vi "Send Inline Buffer.vi"(8 "error in (no error)":errorcluster, 10 "Inline Buffer Parameters":T1, 11 "Dispatcher Interface in":refnum<class "Dispatcher Interface.lvclass">) -> (0 "error out":errorcluster, 3 "Dispatcher Interface out":refnum<class "Dispatcher Interface.lvclass">)   [LabVIEW 2017, in "DSF Core.lvlib" / "Dispatcher Interface.lvclass"]
uses:
  Dispatcher Interface.lvclass
  Inline Buffer Parameters.ctl
  Command Data.ctl
  Command.ctl
  Parameters.ctl
  Write Dispatcher Command.vi
  Interface.lvclass
  Response.ctl
  C:/Git/DSF/Core/Classes/Interface/Interface.lvclass
  Invalid Response.vi
  Invalid Response Parameters.vi
  Read Dispatcher Response.vi
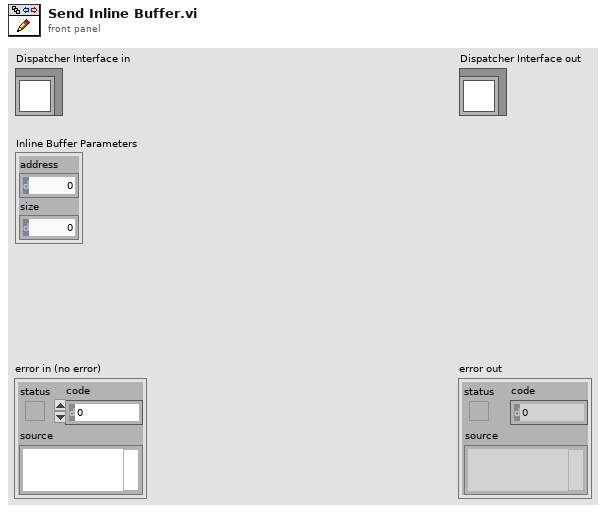
[diagram p1: front panel]
types:
  T1 = typedef "DSF Core.lvlib/Dispatcher Interface.lvclass/Inline Buffer Parameters.ctl" = cluster{"address":u64, "size":u64}
  T2 = typedef "DSF Core.lvlib/Dispatcher Interface.lvclass/Command.ctl" = enum8{"Idle", "Start", "Rx", "Tx", "Set Inline Buffer", "Shutdown", "Error"}
  T3 = typedef "DSF Core.lvlib/Dispatcher Interface.lvclass/Parameters.ctl" = cluster{"arg1":u64, "arg2":u64}
  T4 = typedef "DSF Core.lvlib/Dispatcher Interface.lvclass/Command Data.ctl" = cluster{"Command":T2, "Parameters":T3}
  T5 = typedef "DSF Core.lvlib/Dispatcher Interface.lvclass/Response.ctl" = enum8{"General Ack", "Error", "Shutting Down"}
  T6 = typedef "DSF Core.lvlib/Dispatcher Interface.lvclass/Response Data.ctl" = cluster{"Response":T5, "Parameters":T3}
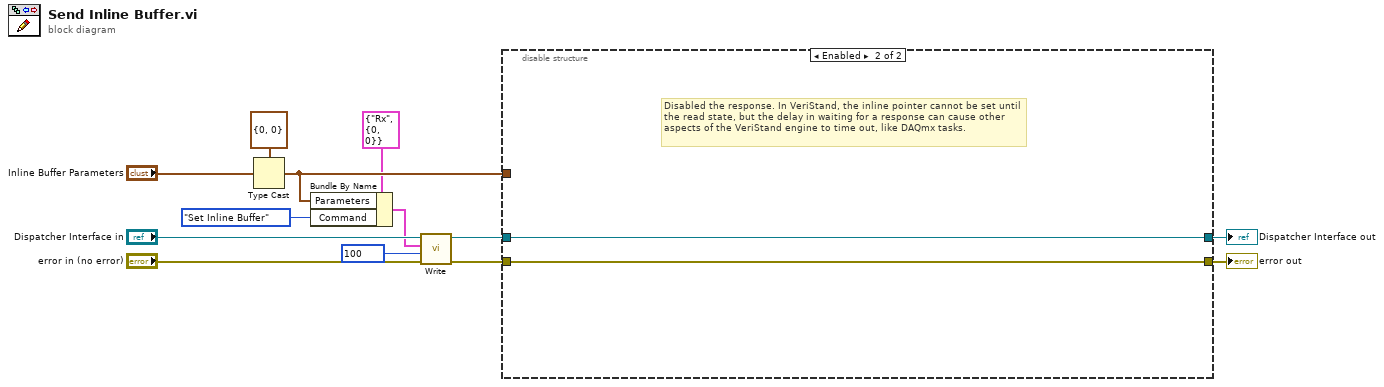
[diagram p0: block diagram]
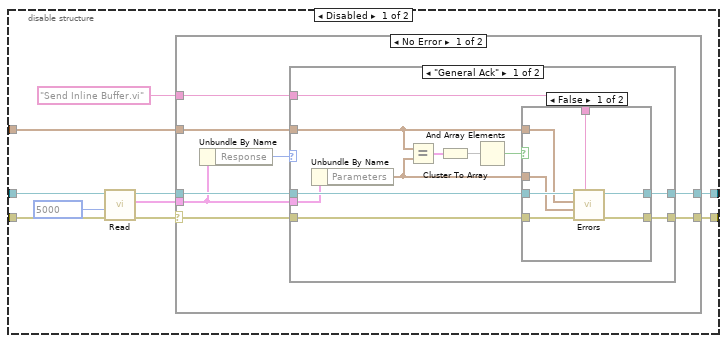
[diagram p2: hidden frame]
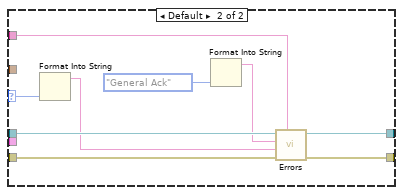
[diagram p4: hidden frame]
diagram:
  n1 = Type Cast(type=T3 {"arg1"=0, "arg2"=0} ("Parameters"), x="Inline Buffer Parameters") -> (*(type *) &x=w5:T3)
  n2 = Bundle By Name(cluster=T4 {"Command"=enum."Rx", "Parameters"={"arg1"=0, "arg2"=0}} ("command"), "Parameters"=w5, "Command"=Command."Set Inline Buffer") -> (w7:T4)
  n3 = call-poly "Write.vi"("error in (no error)"="error in (no error)", "timeout in ms (0)"=100, "command"=w7, "Dispatcher Interface in"="Dispatcher Interface in") -> ("error out"=w3:errorcluster, "Dispatcher Interface out"=w4:refnum<class "Dispatcher Interface.lvclass">)  [unwired: 6 in]
  n4 = disable-structure shown="Enabled" {
    disable-tunnel: [w23 w63] -> w11
    disable-tunnel: [w22 w64] -> w10
    disable-tunnel: w5 -> [w18 _]
    disable-tunnel: w4 -> [w17 w64]
    disable-tunnel: w3 -> [w16 w63]
    frame Disabled {
      n5 = call-poly "Read.vi"("error in (no error)"=w16, "timeout in ms (0)"=5000, "Dispatcher Interface in"=w17) -> ("error out"=w15:errorcluster, "response"=w19:T6, "Dispatcher Interface out"=w21:refnum<class "Dispatcher Interface.lvclass">)  [unwired: 5 in, 1 out]
      n6 = case shown="No Error" w15 {
        selector: w15 -> [w25 w61]
        tunnel: [w30 w61] -> w23
        tunnel: w18 -> [w29 _]
        tunnel: w21 -> [w28 w62]
        tunnel: [w27 w62] -> w22
        tunnel: w19 -> [w26 _]
        tunnel: "Send Inline Buffer.vi" ("error source vi name") -> [w24 _]
        frame No Error {
          n7 = Unbundle By Name(w26) -> ("Response"=w31:T5)
          n8 = case shown="\"General Ack\"" w31 {
            selector: w31 -> [_ w55]
            tunnel: w25 -> [w39 w59]
            tunnel: [w37 w57] -> w30
            tunnel: w29 -> [w34 _]
            tunnel: w28 -> [w36 w60]
            tunnel: [w38 w58] -> w27
            tunnel: w26 -> [w35 _]
            tunnel: w24 -> [w32 w56]
            frame "General Ack" {
              n9 = Unbundle By Name(w35) -> ("Parameters"=w33:T3)
              n10 = Equal?(x=w34, y=w33) -> (x = y?=w42:cluster{"arg1":bool, "arg2":bool})
              n11 = Cluster To Array(cluster=w42) -> (array=w41:bool[])
              n12 = And Array Elements(Boolean array=w41) -> (logical AND=w40:bool)
              n13 = case shown="False" w40 {
                tunnel: w39 -> [w48 w50]
                tunnel: w36 -> [w49 w51]
                tunnel: [w47 w51] -> w38
                tunnel: [w46 w50] -> w37
                tunnel: w34 -> [w44 _]
                tunnel: w33 -> [w45 _]
                tunnel: w32 -> [w43 _]
                frame False {
                  n14 = call-poly "Errors.vi"("error source vi name"=w43, "error in (no error)"=w48, "actual parameters"=w45, "expected parameters"=w44, "Interface in"=w49) -> ("error out"=w46:errorcluster, "Interface out"=w47:refnum<class "Dispatcher Interface.lvclass">)  [unwired: 5 in]
                }
                frame True {
                }
              }
            }
            frame Default {
              n15 = Format Into String(w55) -> (resulting string=w54:string)  [unwired: 3 in, 1 out]
              n16 = Format Into String(Response."General Ack" ("expected response")) -> (resulting string=w52:string)  [unwired: 3 in, 1 out]
              n17 = call-poly "Errors.vi"("error source vi name"=w56, "error in (no error)"=w59, "actual response"=w54, "expected response"=w52, "Interface in"=w60) -> ("error out"=w57:errorcluster, "Interface out"=w58:refnum<class "Dispatcher Interface.lvclass">)  [unwired: 5 in]
            }
          }
        }
        frame Error {
          # "Incoming error. Pass through."
        }
      }
    }
    frame Enabled {
      # "Disabled the response. In VeriStand, the inline pointer cannot be set until the read state, but the delay in waiting for a response can cause other aspects of the VeriStand engine to time out, like DAQmx tasks."
    }
  }
  "error out" <- w11
  "Dispatcher Interface out" <- w10
